vi "RunLoadPeelData.vi"   [LabVIEW 2012]
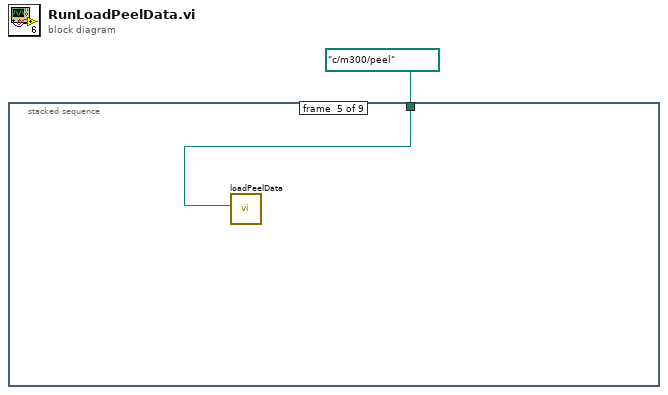
[diagram p0: block diagram]
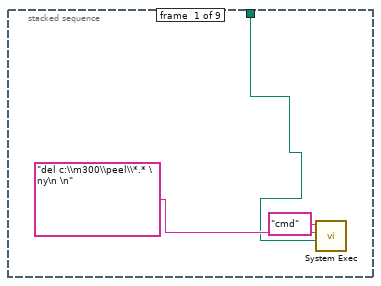
[diagram p2: hidden frame]
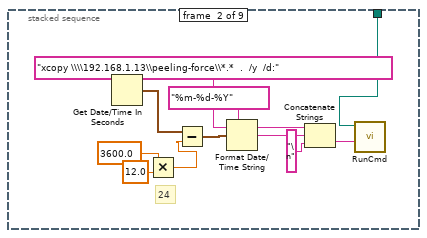
[diagram p3: hidden frame]
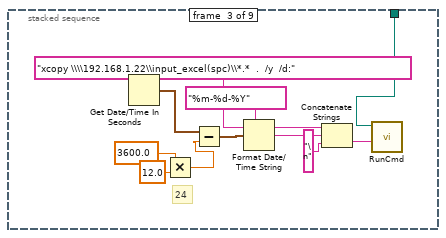
[diagram p4: hidden frame]
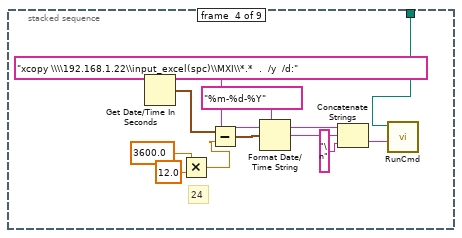
[diagram p5: hidden frame]
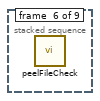
[diagram p6: hidden frame]
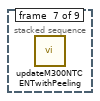
[diagram p7: hidden frame]
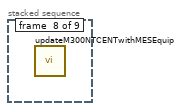
[diagram p8: hidden frame]
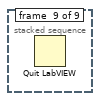
[diagram p9: hidden frame]
diagram:
  n1 = stacked-sequence {
    tunnel: path "c:/m300/peel" ("working directory") -> [w2 w5 w16 w27 w38 _ _ _ _]
    frame #0 {
      n2 = call <vilib>:"System Exec.vi"("working directory"=w2, "standard input"="del c:\\m300\\peel\\*.* \ny\n \n" ("Cmd String"), "command line"="cmd") -> ()  [unwired: 5 in, 4 out]
    }
    frame #1 {
      # "24"
      n3 = Get Date/Time In Seconds() -> (seconds since 1Jan1904=w6:timestamp)
      n4 = Multiply(x=3600.0, y=12.0) -> (x*y=w8:dbl)
      n5 = Subtract(x=w6, y=w8) -> (x-y=w9:timestamp)
      n6 = Format Date/Time String(time format string (%c)="%m-%d-%Y", seconds (now)=w9) -> (date/time string=w12:string)  [unwired: 1 in]
      n7 = Concatenate Strings("xcopy \\\\192.168.1.13\\peeling-force\\*.*  .  /y  /d:" ("string"), w12, "\n" ("string")) -> (w15:string)
      n8 = call "RunCmd.vi"("Cmd String"=w15, "working directory"=w5) -> ()  [unwired: 8 in, 2 out]
    }
    frame #2 {
      # "24"
      n9 = Get Date/Time In Seconds() -> (seconds since 1Jan1904=w17:timestamp)
      n10 = Multiply(x=3600.0, y=12.0) -> (x*y=w19:dbl)
      n11 = Subtract(x=w17, y=w19) -> (x-y=w20:timestamp)
      n12 = Format Date/Time String(time format string (%c)="%m-%d-%Y", seconds (now)=w20) -> (date/time string=w23:string)  [unwired: 1 in]
      n13 = Concatenate Strings("xcopy \\\\192.168.1.22\\input_excel(spc)\\*.*  .  /y  /d:" ("string"), w23, "\n" ("string")) -> (w26:string)
      n14 = call "RunCmd.vi"("Cmd String"=w26, "working directory"=w16) -> ()  [unwired: 8 in, 2 out]
    }
    frame #3 {
      # "24"
      n15 = Get Date/Time In Seconds() -> (seconds since 1Jan1904=w28:timestamp)
      n16 = Multiply(x=3600.0, y=12.0) -> (x*y=w30:dbl)
      n17 = Subtract(x=w28, y=w30) -> (x-y=w31:timestamp)
      n18 = Format Date/Time String(time format string (%c)="%m-%d-%Y", seconds (now)=w31) -> (date/time string=w34:string)  [unwired: 1 in]
      n19 = Concatenate Strings("xcopy \\\\192.168.1.22\\input_excel(spc)\\MXI\\*.*  .  /y  /d:" ("string"), w34, "\n" ("string")) -> (w37:string)
      n20 = call "RunCmd.vi"("Cmd String"=w37, "working directory"=w27) -> ()  [unwired: 8 in, 2 out]
    }
    frame #4 {
      n21 = call "loadPeelData.vi"("path"=w38) -> ()  [unwired: 11 in]
    }
    frame #5 {
      n22 = call "peelFileCheck.vi"() -> ()  [unwired: 12 in]
    }
    frame #6 {
      n23 = call "updateM300NTCENTwithPeeling.vi"() -> ()  [unwired: 12 in]
    }
    frame #7 {
      n24 = call "updateM300NTCENTwithMESEquip.vi"() -> ()  [unwired: 12 in]
    }
    frame #8 {
      n25 = Quit LabVIEW() -> ()  [unwired: 1 in]
    }
  }
